vi "CloseListener.vi"(8 "error in (no error)":errorcluster, 11 "WebSocket in":refnum<class "WebSocket.lvclass">) -> (0 "error out":errorcluster, 3 "WebSocket out":refnum<class "WebSocket.lvclass">)   [LabVIEW 2019, in "WebSocket.lvlib" / "WebSocket.lvclass"]
uses:
  WebSocket.lvclass
  WebSocket.lvclass/WebSocket.ctl
  <vilib>/MediaMongrels Ltd/WebSockets/Sockets/VISA TCP Listener/VISA TCP Listener.lvclass
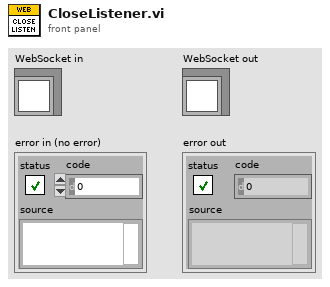
[diagram p1: front panel]
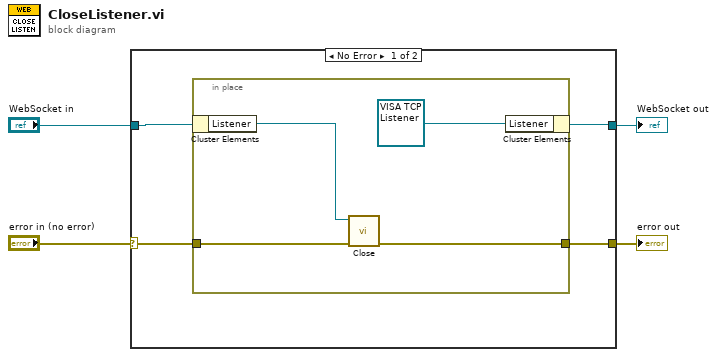
[diagram p0: block diagram]
diagram:
  n1 = case shown="No Error" "error in (no error)" {
    selector: "error in (no error)" -> [w7 w14]
    tunnel: [w6 w14] -> w3
    tunnel: [w5 w13] -> w1
    tunnel: "WebSocket in" -> [w8 w13]
    frame No Error {
      n2 = in-place {
        in-place-border: w7 -> [w11]
        in-place-border: [w10] -> w6
        n3 = in-place-cluster #1(w8) -> ("Listener"=w12:refnum<class "VISA TCP Listener.lvclass">)
        n4 = call-dynamic "Close.vi"("error in (no error)"=w11, "VISA TCP Listener in"=w12) -> ("error out"=w10:errorcluster)  [unwired: 9 in]
        n5 = in-place-cluster #1("Listener"=refnum<class "VISA TCP Listener.lvclass"> refnum ("VISA TCP Listener out")) -> (w5:refnum<class "WebSocket.lvclass">)
      }
    }
    frame Error {
    }
  }
  "error out" <- w3
  "WebSocket out" <- w1
